vi "DI N Samples（Host）.vi"() -> ()   [LabVIEW 2019]
uses:
  <vilib>/FPGAPlugInAG/ELVIS III/niLvFpga_Open_ELVIS III.vi
  <vilib>/rvi/interface/common/dynamic/niFpgaDynamicAddResources.vi
  <vilib>/rvi/interface/common/niFpgaWaitOnOcc.vi
  <vilib>/Utility/error.llb/Error Cluster From Error Code.vi
  <vilib>/FPGAPlugInAG/Dynamic/niLvFpga_Run_Dynamic.vi
  <vilib>/rvi/errors/niLvFpgaAdjustHostInterfaceError.vi
  <vilib>/FPGAPlugInAG/Dynamic/niLvFpga_Close_Dynamic.vi
  <vilib>/rvi/interface/nirviOpenFPGA/nirviOpenFPGA.xnode
  FPGA Bitfiles/analogio-fpga_FPGATarget_DINSamples_5-+ly1nIZhU.lvbitx
  DI N Samples.vi
  <vilib>/rvi/interface/nirviMethod/nirviMethod.xnode
  <vilib>/rvi/interface/nirviReadWriteControl/nirviReadWriteControl.xnode
  <vilib>/rvi/interface/nirviCloseFPGA/nirviCloseFPGA.xnode
  NiFpgaLv.dll
  <vilib>/rvi/interface/Simulation/niFpgaSimulationCallBeginRW.vi
  <vilib>/FPGAPlugInAG/Dynamic/niLvFpga_ConfigureFifo_Dynamic.vi
  <vilib>/rvi/errors/niLvFpgaMergeErrorWithErrorCode.vi
  <vilib>/FPGAPlugInAG/Dynamic/niLvFpga_ReadFifo_Dynamic.vi
panel:
  out "数字波形图 2":digitalwaveform(graph)
  out "数字波形图":digitalwaveform(graph)
  in  "停止":bool
  in  "DI.B.DMA_ENA":bool
  in  "DI.A.DMA_ENA":bool
  in  "DI.B.DMA_CNTR":u16
  in  "DI.A.DMA_CNTR":u16
  in  "B.DIR":bool[](array[boolean])
  in  "A.DIR":bool[](array[boolean])
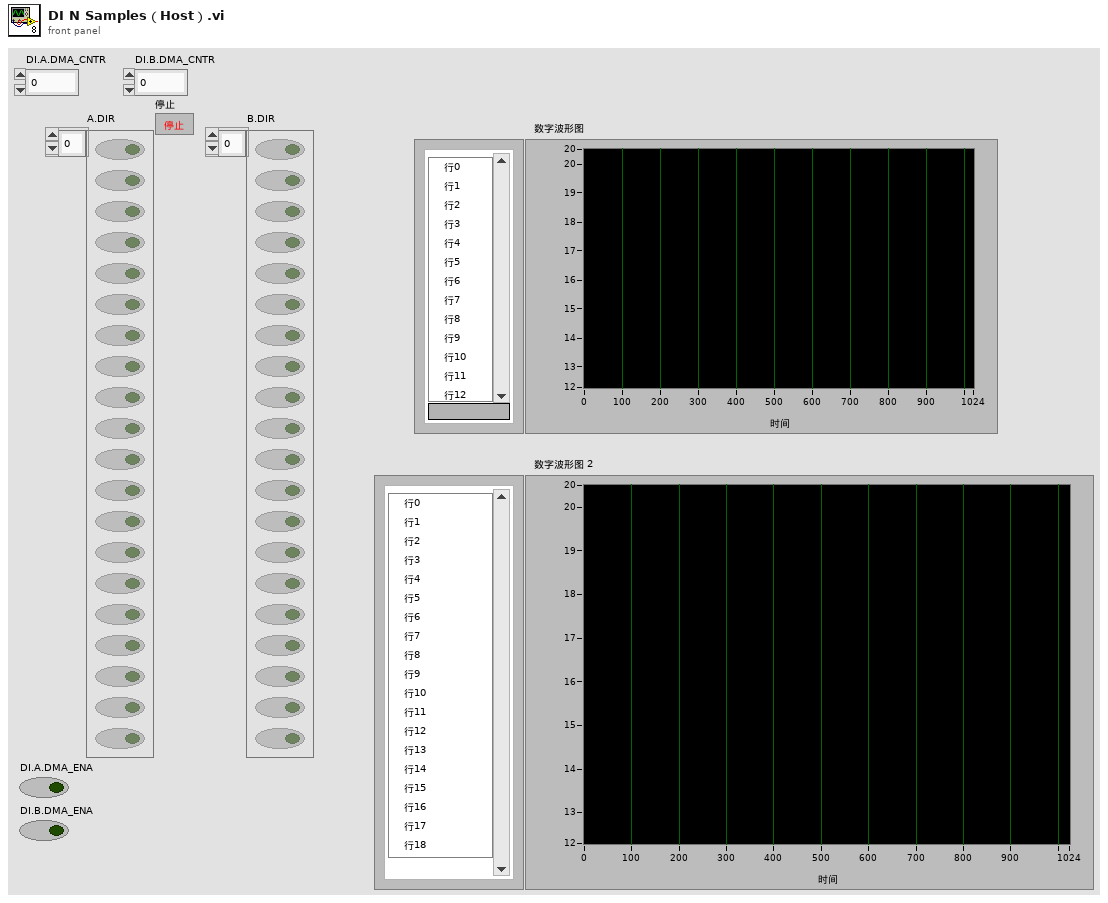
[diagram p1: front panel]
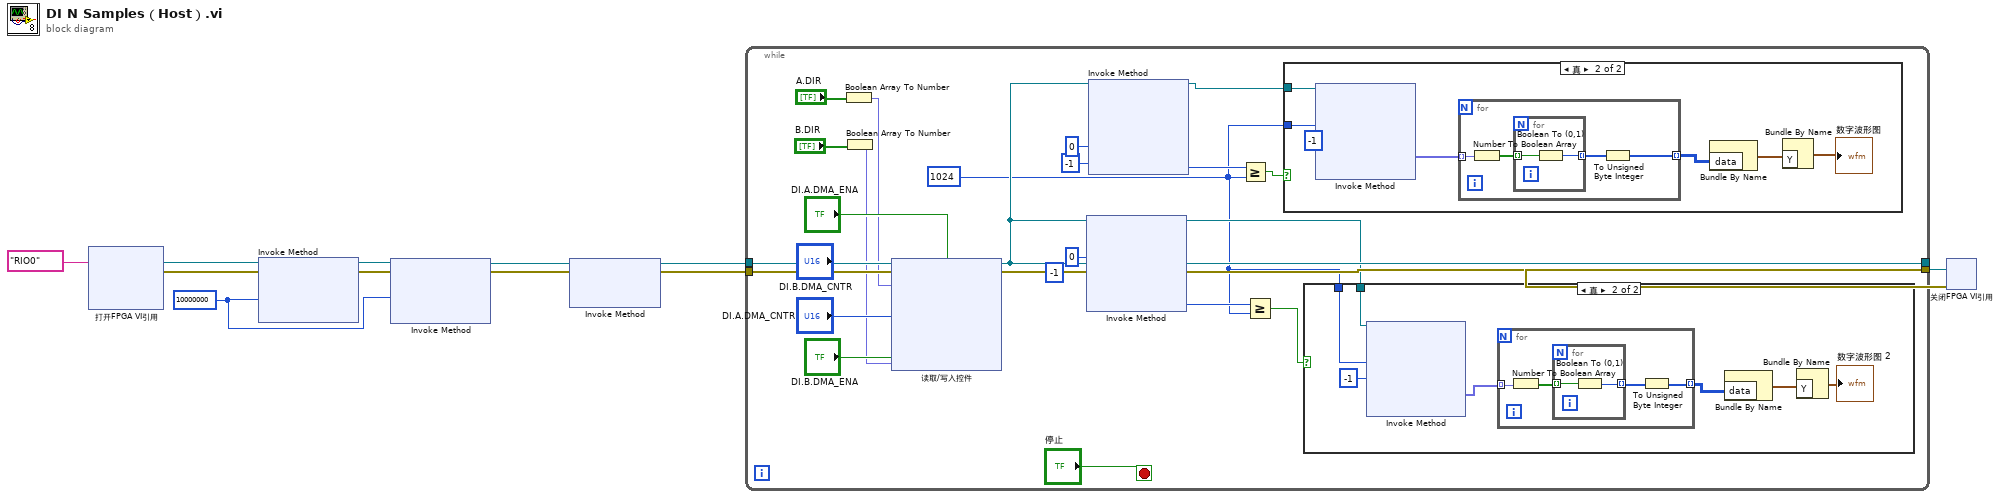
[diagram p0: block diagram]
diagram:
  w1 = u32 10000000 ("请求的深度")
  n1 = xnode "打开FPGA VI引用"("资源名称"=tag "RIO0") -> ("FPGA VI引用输出"=w8:refnum<k20>, "错误输出"=w9:errorcluster)  [unwired: 1 in]
  n2 = xnode "Invoke Method"("FPGA VI引用输入"=w8, "错误输入"=w9, "请求的深度"=w1) -> ("FPGA VI引用输出"=w6:refnum<k20>, "错误输出"=w7:errorcluster)  [unwired: 1 out]
  n3 = xnode "Invoke Method"("FPGA VI引用输入"=w6, "错误输入"=w7, "请求的深度"=w1) -> ("FPGA VI引用输出"=w4:refnum<k20>, "错误输出"=w5:errorcluster)  [unwired: 1 out]
  n4 = xnode "Invoke Method"("FPGA VI引用输入"=w4, "错误输入"=w5) -> ("FPGA VI引用输出"=w2:refnum<k20>, "错误输出"=w3:errorcluster)  [unwired: 1 in]
  n5 = while {
    tunnel: w3 -> [w36]
    tunnel: w2 -> [w35]
    tunnel: [w25] -> w10
    tunnel: [w22] -> w11
    stop <- "停止" stop-if-true
    w13 = u32 1024 ("y")
    n6 = Boolean Array To Number ("布尔数组至数值转换")(Boolean array="A.DIR") -> (number=w28:fxp<+,20,20>)
    n7 = Boolean Array To Number ("布尔数组至数值转换")(Boolean array="B.DIR") -> (number=w27:fxp<+,20,20>)
    n8 = xnode "读取/写入控件"("FPGA VI引用输入"=w35, "错误输入"=w36, "DIO.A_19:0.DIR"=w28, "DI.A.DMA_ENA"="DI.A.DMA_ENA", "DI.A.DMA_CNTR"="DI.A.DMA_CNTR", "DI.B.DMA_CNTR"="DI.B.DMA_CNTR", "DI.B.DMA_ENA"="DI.B.DMA_ENA", "DIO.B_19:0.DIR"=w27) -> ("FPGA VI引用输出"=w22:refnum<k20>, "错误输出"=w25:errorcluster)
    n9 = xnode "Invoke Method"("FPGA VI引用输入"=w22, "元素数量"=u32 0, "超时(ms)"=-1) -> ("FPGA VI引用输出"=w14:refnum<k20>, "剩余元素"=w18:u32)  [unwired: 1 in, 2 out]
    n10 = xnode "Invoke Method"("FPGA VI引用输入"=w22, "元素数量"=u32 0, "超时(ms)"=-1) -> ("FPGA VI引用输出"=w16:refnum<k20>, "剩余元素"=w19:u32)  [unwired: 1 in, 2 out]
    n11 = Greater Or Equal?(x=w19, y=w13) -> (x >= y?=w17:bool)
    n12 = Greater Or Equal?(x=w18, y=w13) -> (x >= y?=w15:bool)
    n13 = case shown="真" w17 {
      tunnel: w13 -> [_ w56]
      tunnel: w16 -> [_ w54]
      frame False {
      }
      frame True {
        n14 = xnode "Invoke Method"("FPGA VI引用输入"=w54, "元素数量"=w56, "超时(ms)"=-1) -> ("数据"=w53:fxp<+,20,20>[])  [unwired: 1 in, 3 out]
        n15 = for {
          tunnel: w53 -> [w60] mode=indexing
          tunnel: [w57] -> w50 mode=indexing
          n16 = Number To Boolean Array(number=w60) -> (Boolean array=w59:bool[])
          n17 = for {
            tunnel: w59 -> [w62] mode=indexing
            tunnel: [w61] -> w58 mode=indexing
            n18 = Boolean To (0,1)(Boolean=w62) -> (0, 1=w61:i16)
          }
          n19 = To Unsigned Byte Integer(number=w58) -> (unsigned 8bit integer=w57:u8[])
        }
        n20 = Bundle By Name ("创建数字数据")("data"=w50) -> (w51:digitaldata)  [unwired: 1 in]
        n21 = Bundle By Name ("创建波形")("Y"=w51) -> (→"数字波形图":digitalwaveform)  [unwired: 1 in]
      }
    }
    n22 = case shown="真" w15 {
      tunnel: w14 -> [_ w43]
      tunnel: w13 -> [_ w42]
      frame False {
      }
      frame True {
        n23 = xnode "Invoke Method"("FPGA VI引用输入"=w43, "元素数量"=w42, "超时(ms)"=-1) -> ("数据"=w40:fxp<+,20,20>[])  [unwired: 1 in, 3 out]
        n24 = for {
          tunnel: w40 -> [w47] mode=indexing
          tunnel: [w44] -> w38 mode=indexing
          n25 = Number To Boolean Array(number=w47) -> (Boolean array=w46:bool[])
          n26 = for {
            tunnel: w46 -> [w49] mode=indexing
            tunnel: [w48] -> w45 mode=indexing
            n27 = Boolean To (0,1)(Boolean=w49) -> (0, 1=w48:i16)
          }
          n28 = To Unsigned Byte Integer(number=w45) -> (unsigned 8bit integer=w44:u8[])
        }
        n29 = Bundle By Name ("创建数字数据")("data"=w38) -> (w39:digitaldata)  [unwired: 1 in]
        n30 = Bundle By Name ("创建波形")("Y"=w39) -> (→"数字波形图 2":digitalwaveform)  [unwired: 1 in]
      }
    }
  }
  n31 = xnode "关闭FPGA VI引用"("FPGA VI引用输入"=w11, "错误输入"=w10) -> ()  [unwired: 1 out]
